vi "File HDF5 Write.vi"(9 "Timestamp":u64[](array[numeric]), 10 "BPM and PS Data":dbl[][](array[numeric]), 11 "HDF IDs in":T1) -> (3 "Array":i32[](array[numeric]))   [LabVIEW 2011]
uses:
  Types Definitions/Type HDF IDs.ctl
  <instrlib>/Soft Front Panel File/sfpFile.llb/sfpFile Extend DBL Vector.vi
panel:
  out "error out":errorcluster
  in  "error in (no error)":errorcluster
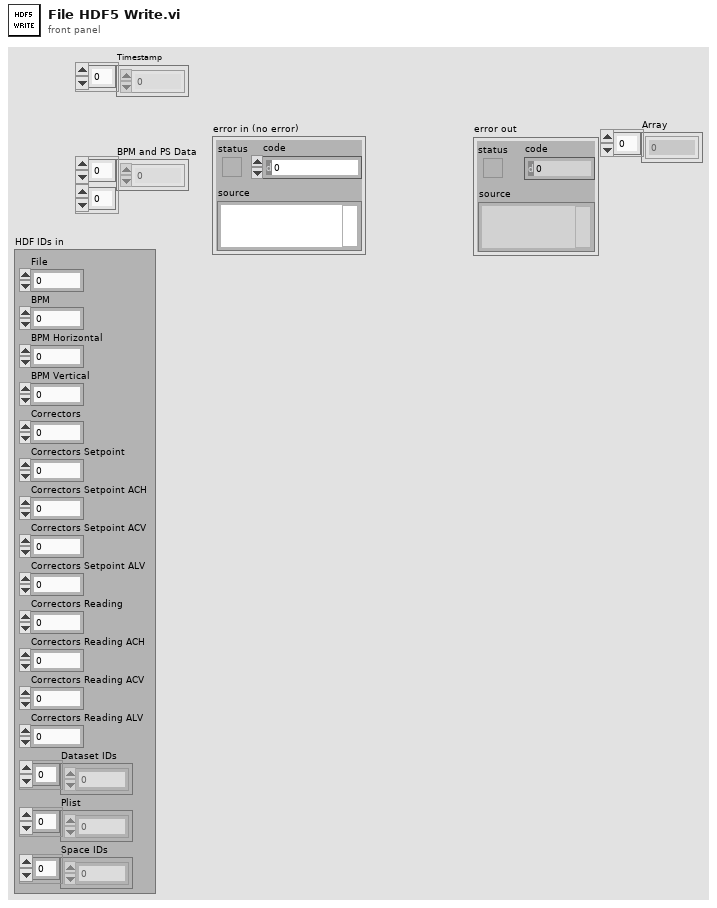
[diagram p1: front panel]
types:
  T1 = typedef "Type HDF IDs.ctl" = cluster{"File":i32, "BPM":i32, "BPM Horizontal":i32, "BPM Vertical":i32, "Correctors":i32, "Correctors Setpoint":i32, "Correctors Setpoint ACH":i32, "Correctors Setpoint ACV":i32, "Correctors Setpoint ALV":i32, "Correctors Reading":i32, "Correctors Reading ACH":i32, "Correctors Reading ACV":i32, "Correctors Reading ALV":i32, "Dataset IDs":i32[], "Plist":i32[], "Space IDs":i32[]}
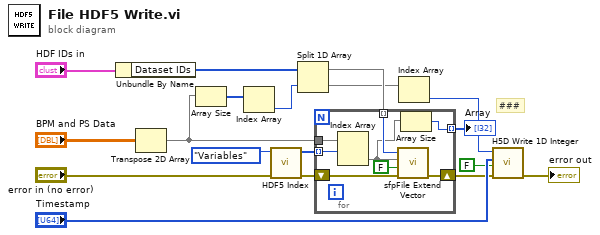
[diagram p0: block diagram]
diagram:
  # "###"
  n1 = Unbundle By Name("HDF IDs in") -> ("Dataset IDs"=w17:i32[])
  n2 = Transpose 2D Array(2D array="BPM and PS Data") -> (transposed array=w9:dbl[][])
  n3 = Array Size(array=w9) -> (size(s)=w13:i32[])
  n4 = Index Array(array=w13) -> (element=w8:i32)  [unwired: 1 in]
  n5 = call "HDF5 Index.vi"("error in (no error)"="error in (no error)", "Mapping Type"=enum16{"Dataset", "Variables"}."Variables") -> ("error out"=w14:errorcluster, "Mapping out"=w11:i32[])  [unwired: 8 in]
  n6 = Split 1D Array(array=w17, index=w8) -> (first subarray=w16:i32[], second subarray=w15:i32[])
  n7 = for {
    tunnel: w11 -> [w26] mode=indexing
    tunnel: w9 -> [w25]
    tunnel: w16 -> [w21] mode=indexing
    shift-right: [w24] -> w4
    shift-left: w14 -> [w23]
    tunnel: [w19] -> w1 mode=indexing
    n8 = Index Array(array=w25, index (row)=w26) -> (element=w20:dbl[])  [unwired: 1 in]
    n9 = call-poly <instrlib>:"sfpFile Extend Vector.vi"("error in (no error)"=w23, "close?"=FALSE, "new data"=w20, "dataset_id"=w21) -> ("error out"=w24:errorcluster)  [unwired: 6 in, 1 out]
    n10 = Array Size(array=w20) -> (size(s)=w19:i32)
  }
  "Array" <- w1
  n11 = Index Array(array=w15) -> (element=w6:i32)  [unwired: 1 in]
  n12 = call "H5D Write 1D Integer.vi"("error in (no error)"=w4, "close?"=FALSE, "new data"="Timestamp", "dataset_id"=w6) -> ("error out"=→"error out":errorcluster)  [unwired: 6 in, 1 out]
